vi "BB_Image_Process.vi"(8 "Use Calibration":bool=TRUE, 9 "Color Controls":T3={"Hue"={107.81818389892578, 139.81818389892578}, "Sat"={176.07142857142858, 255.0}, "Val"={40.53571428571429, 255.0}} {"Hue" scale=0.0..255.0 scale format="%#_3g"}, 10 "Mask":T2, 11 "Input Image":T2) -> (1 "Results":T4 {"Score" format="%#_3g"; "Pixels"."Rectangle"."Numeric 5" format="%#_3g"; "Pixels"."Rectangle"."Numeric 3" format="%#_3g"; "Pixels"."Rectangle"."Numeric 2" format="%#_3g"; "Pixels"."Rectangle"."Numeric" format="%#_3g"; "Normalized"."Rectangle"."Numeric 5" format="%#_2g"; "Normalized"."Rectangle"."Numeric 3" format="%#_2g"; "Normalized"."Rectangle"."Numeric 2" format="%#_2g"; "Normalized"."Rectangle"."Numeric" format="%#_2g"; "Normalized"."Center"."?" format="%#_3g"; "Normalized"."Center"."?" format="%#_3g"; "Distance (ft)" format="%#_3g"}, 2 "Mask":T2(plugin-control), 3 "Original Image":T2(plugin-control))   [LabVIEW 2016]
uses:
  Vision Support Code/Camera Types.ctl
  <vilib>/vision/Image Controls.llb/IMAQ Image.ctl
  <vilib>/vision/NI_Vision_Development_Module.lvlib
panel:
  in  "Dilate":bool=TRUE
  in  "Operation 2":T1(ring)=enum."Erode"
  in  "Operation":T1(ring)=enum."Dilate"
  in  "Number of iterations (1) 2":i32=1
  in  "Number of iterations (1)":i32=1
  out "Qualified Particles":i32
  in  "Annotate":bool=TRUE
  in  "Camera Type":T5=enum."MS HD3000 square"
  in  "Score Cutoff %":dbl=70.0
  in  "Particles":dbl=5.0
  in  "Color Mode":u16(ring)=3 items=["RGB", "HSL", "HSV", "HSI"]
  in  "Line Border":cluster{"Top":dbl, "Bottom":dbl}={"Top"=6.0, "Bottom"=1.0}
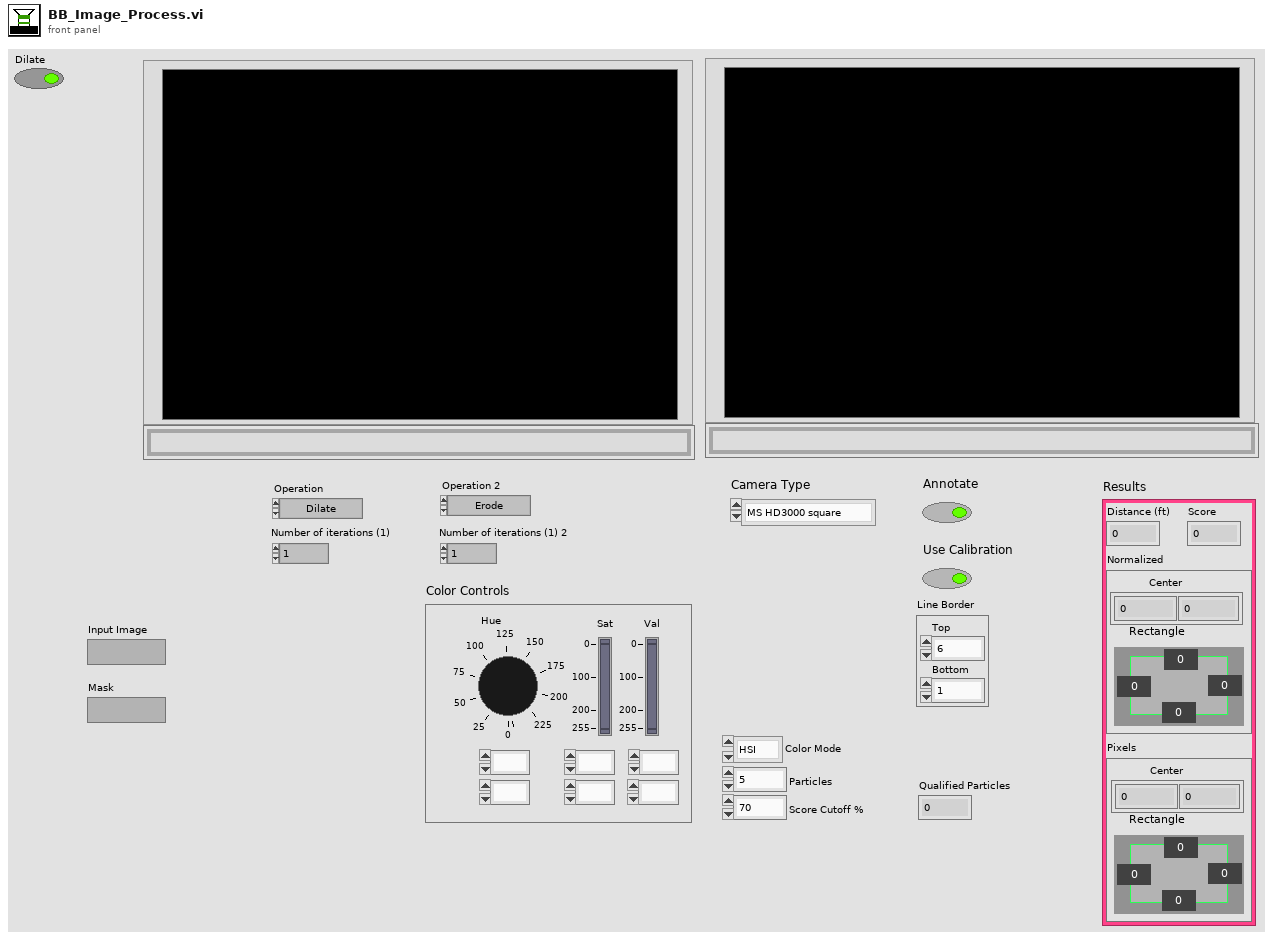
[diagram p1: front panel]
types:
  T1 = enum32{"AutoM", "Close", "Dilate", "Erode", "Gradient", "Gradient out", "Gradient in", "Hit miss", "Open", "PClose", "POpen", "Thick", "Thin"}
  T2 = typedef "IMAQ Image.ctl" = refnum<image>
  T3 = cluster{"Hue":cluster{dbl, dbl}, "Sat":cluster{dbl, dbl}, "Val":cluster{dbl, dbl}}
  T4 = cluster{"Distance (ft)":dbl, "Score":dbl, "Normalized":cluster{"Center":cluster{dbl, dbl}, "Rectangle":cluster{"Numeric":dbl, "Numeric 2":dbl, "Numeric 3":dbl, "Numeric 5":dbl}}, "Pixels":cluster{"Center":cluster{dbl, dbl}, "Rectangle":cluster{"Numeric":dbl, "Numeric 2":dbl, "Numeric 3":dbl, "Numeric 5":dbl}}}
  T5 = typedef "Camera Types.ctl" = enum16{"206", "1011", "1013", "MS HD3000 square", "MS HD3000 640x480"}
  T6 = typedef "Image Type" = u32
  T7 = typedef "Particle Parameters" = i32
  T8 = cluster{"Left":dbl, "Top":dbl, "Right":dbl, "Bottom":dbl}
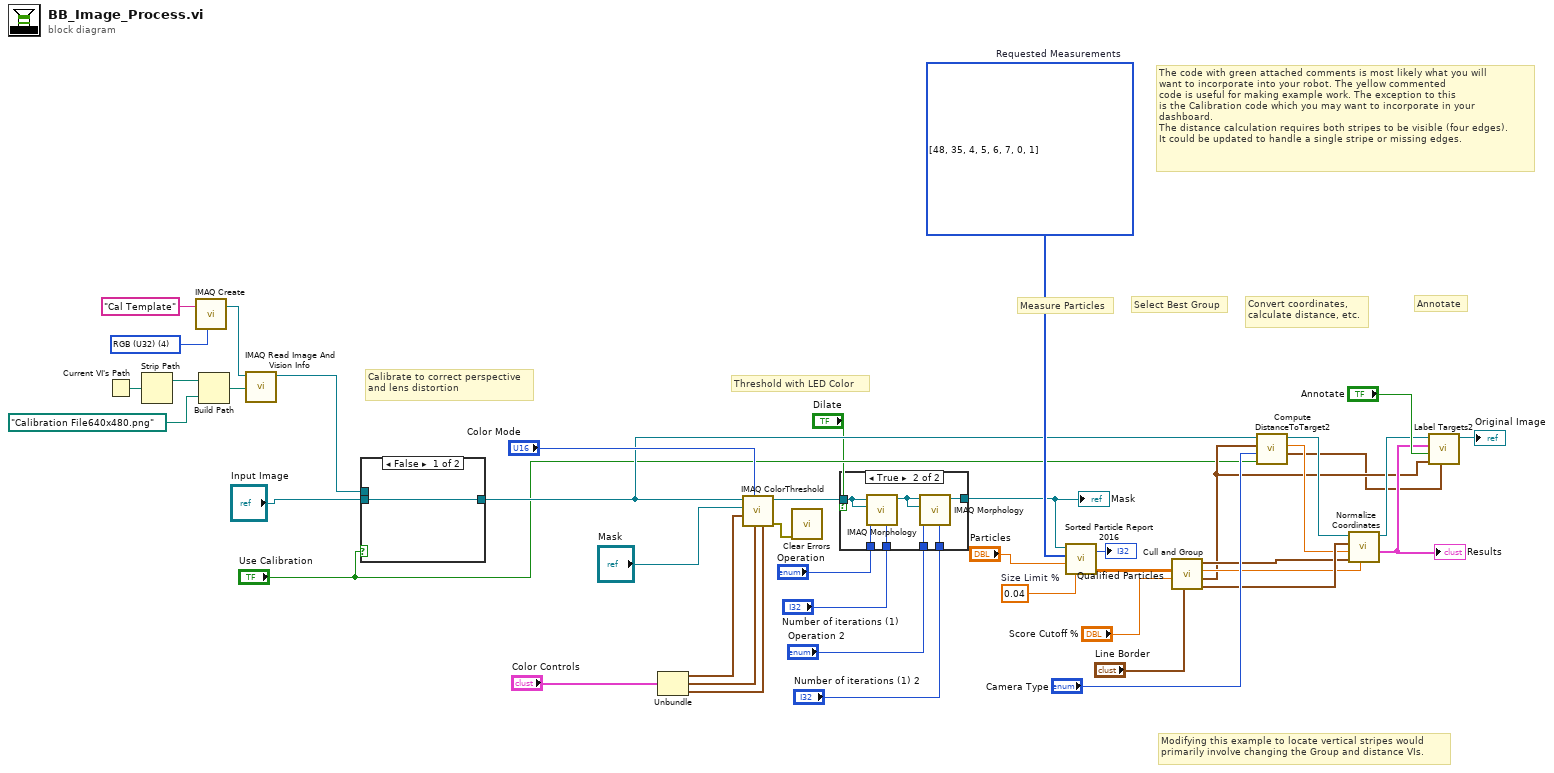
[diagram p0: block diagram]
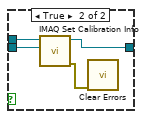
[diagram p3: hidden frame]
diagram:
  w31 = 0.04  # Size Limit %
  w43 = T6 4 items=["Grayscale (U8)", "Grayscale (I16)", "Grayscale (SGL)", "Complex (CSG)", "RGB (U32)", "HSL (U32)", "RGB (U64)", "Grayscale (U16)"] ("Image Type")
  w44 = T7[] [48, 35, 4, 5, 6, 7, 0, 1] items=["Center of Mass X", "Center of Mass Y", "First Pixel X", "First Pixel Y", "Bounding Rect Left", "Bounding Rect Top", "Bounding Rect Right", "Bounding Rect Bottom", "Max Feret Diameter Start X", "Max Feret Diameter Start Y", "Max Feret Diameter End X", "Max Feret Diameter End Y", "Max Horiz. Segment Length Left", "Max Horiz. Segment Length Right", "Max Horiz. Segment Length Row", "-", "Bounding Rect Width", "Bounding Rect Height", "Bounding Rect Diagonal", "Perimeter", "Convex Hull Perimeter", "Holes' Perimeter", "Max Feret Diameter", "Equivalent Ellipse Major Axis", "Equivalent Ellipse Minor Axis", "Equivalent Ellipse Minor Axis (Feret)", "Equivalent Rect Long Side", "Equivalent Rect Short Side", "Equivalent Rect Diagonal", "Equivalent Rect Short Side (Feret)", "Average Horiz. Segment Length", "Average Vert. Segment Length", "Hydraulic Radius", "Waddel Disk Diameter", "-", "Area", "Holes' Area", "Particle & Holes' Area", "Convex Hull Area", "Image Area", "-", "Number of Holes", "Number of Horiz. Segments", "Number of Vert. Segments", "-", "Orientation", "Max Feret Diameter Orientation", "-", "% Area/Image Area", "% Area/(Particle & Holes' Area)", "Ratio of Equivalent Ellipse Axes", "Ratio of Equivalent Rect Sides", "-", "Elongation Factor", "Compactness Factor", "Heywood Circularity Factor", "Type Factor", "-", "Sum X", "Sum Y", "Sum XX", "Sum XY", "Sum YY", "Sum XXX", "Sum XXY", "Sum XYY", "Sum YYY", "-", "Moment of Inertia XX", "Moment of Inertia XY", "Moment of Inertia YY", "Moment of Inertia XXX", "Moment of Inertia XXY", "Moment of Inertia XYY", "Moment of Inertia YYY", "Norm. Moment of Inertia XX", "Norm. Moment of Inertia XY", "Norm. Moment of Inertia YY", "Norm. Moment of Inertia XXX", "Norm. Moment of Inertia XXY", "Norm. Moment of Inertia XYY", "Norm. Moment of Inertia YYY", "Hu Moment 1", "Hu Moment 2", "Hu Moment 3", "Hu Moment 4", "Hu Moment 5", "Hu Moment 6", "Hu Moment 7"]  # Requested Measurements
  # "Calibrate to correct perspective\nand lens distortion"
  # "Measure Particles"
  # "Convert coordinates,\ncalculate distance, etc."
  # "Annotate"
  # "Select Best Group"
  # "Threshold with LED Color"
  # "Modifying this example to locate vertical stripes would\nprimarily involve changing the Group and distance VIs."
  # "The code with green attached comments is most likely what you will\nwant to incorporate into your robot. The yellow commented\ncode is useful for making example work. The exception to this\nis the Calibration code which you may want to incorporate in your\ndashboard.\nThe distance calculation requires both stripes to be visible (four edges).\nIt could be updated to handle a single stripe or missing edges."
  n1 = Current VI's Path() -> (path=w39:path)
  n2 = Strip Path(path=w39) -> (stripped path=w36:path)  [unwired: 1 out]
  n3 = call "IMAQ Create"("Image Name"="Cal Template", "Image Type"=w43) -> ("New Image"=w41:T2)  [unwired: 2 in, 2 out]
  n4 = Build Path(base path=w36, name or relative path=path "Calibration File640x480.png" ("Folder Location")) -> (appended path=w38:path)
  n5 = call "IMAQ Read Image And Vision Info"("File Path"=w38, "Image"=w41) -> ("Image Out"=w40:T2)  [unwired: 7 in, 2 out]
  n6 = case shown="False" "Use Calibration" {
    tunnel: [w45 w49] -> w12
    tunnel: "Input Image" -> [w45 w46]
    tunnel: w40 -> [_ w48]
    frame False {
    }
    frame True {
      n7 = call "IMAQ Set Calibration Info"("Image Dst"=w46, "Image Src"=w48) -> ("error out"=w47:errorcluster, "Calibrated Image"=w49:T2)  [unwired: 8 in]
      n8 = call <vilib>:"Clear Errors.vi"("error in (no error)"=w47) -> ()  [unwired: 5 in, 2 out]
    }
  }
  n9 = Unbundle("Color Controls") -> ("Hue"=w35:cluster{dbl, dbl}, "Sat"=w34:cluster{dbl, dbl}, "Val"=w33:cluster{dbl, dbl})
  n10 = call "IMAQ ColorThreshold"("Blue or Luma or Val or Inten Range"=w33, "Green or Sat Range"=w34, "Color Mode"="Color Mode", "Red or Hue Range"=w35, "Image Dst"="Mask", "Image Src"=w12) -> ("error out"=w28:errorcluster, "Image Dst Out"=w2:T2)  [unwired: 4 in]
  n11 = call <vilib>:"Clear Errors.vi"("error in (no error)"=w28) -> ()  [unwired: 5 in, 2 out]
  n12 = case shown="True" "Dilate" {
    tunnel: "Number of iterations (1)" -> [_ w57]
    tunnel: [w50 w56] -> w6
    tunnel: "Number of iterations (1) 2" -> [_ w55]
    tunnel: "Operation" -> [_ w54]
    tunnel: "Operation 2" -> [_ w53]
    tunnel: w2 -> [w50 w52]
    frame False {
    }
    frame True {
      n13 = call "IMAQ Morphology"("Number of iterations (1)"=w57, "Operation"=w54, "Image Dst"=w52, "Image Src"=w52) -> ("Image Dst Out"=w51:T2)  [unwired: 6 in, 1 out]
      n14 = call "IMAQ Morphology"("Number of iterations (1)"=w55, "Operation"=w53, "Image Dst"=w51, "Image Src"=w51) -> ("Image Dst Out"=w56:T2)  [unwired: 6 in, 1 out]
    }
  }
  "Mask" <- w6
  n15 = call "Sorted Particle Report 2016.vi"("Min Area Size %"=w31, "Particle Count Limit"="Particles", "Pixel Measurements"=w44, "Image in"=w6) -> ("Sorted Data"=w26:dbl[][], "Particles"=→"Qualified Particles":i32)
  n16 = call "Cull and Group.vi"("Line Border"="Line Border", "Score Cutoff"="Score Cutoff %", "Sorted Data"=w26) -> ("Rect"=w23:T8, "Line"=w14:T8, "Score"=w17:dbl, "Center"=w19:cluster{"X":dbl, "Y":dbl})  [unwired: 5 in]
  n17 = call "Compute DistanceToTarget2.vi"("Calibrated"="Use Calibration", "Camera Type"="Camera Type", "Line"=w14, "Image Src"=w12) -> ("Edges"=w13:cluster{"X":sgl, "Y":sgl}[], "Distance (ft)"=w22:dbl, "Image Dst Out"=w21:T2)  [unwired: 5 in]
  n18 = call "Normalize Coordinates.vi"("Score"=w17, "Center"=w19, "Distance"=w22, "Bounding box"=w23, "Image in"=w21) -> ("Results"=w18:T4, "Image out"=w20:T2)  [unwired: 5 in]
  "Results" <- w18
  n19 = call "Label Targets2.vi"("Edges"=w13, "Line"=w14, "Annotate"="Annotate", "Results"=w18, "Image in"=w20) -> ("Image out"=→"Original Image":T2)  [unwired: 6 in]
